vi "TetroInfoModulation.vi"(9 "TetroInfo Input":T1, 10 "GameCommand enum":T2, 11 "Playfield Input":bool[][](array[boolean])) -> (1 "TetroInfo Output":T1)   [LabVIEW 2026]
doc: "This VI i responsible for modifying an existing tetro info according to the users game commands"
uses:
  01_Typen/GameCommandTypeDef.ctl
  02_StateMachine/GameTetrominoInformationTypeDef.ctl
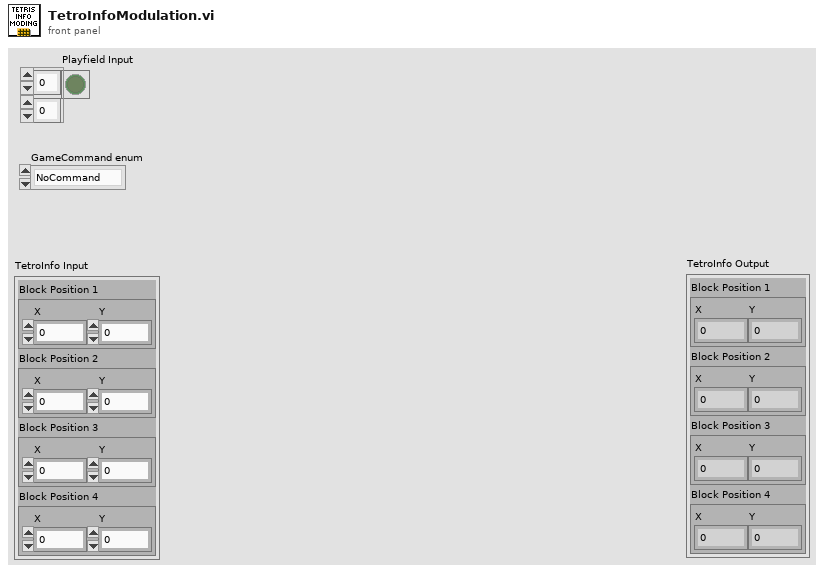
[diagram p1: front panel]
types:
  T1 = typedef "GameTetrominoInformationTypeDef.ctl" = cluster{"Block Position 1":cluster{"X":i32, "Y":i32}, "Block Position 2":cluster{"X":i32, "Y":i32}, "Block Position 3":cluster{"X":i32, "Y":i32}, "Block Position 4":cluster{"X":i32, "Y":i32}}
  T2 = typedef "GameCommandTypeDef.ctl" = enum16{"NoCommand", "Rotate", "MoveLeft", "MoveRight"}
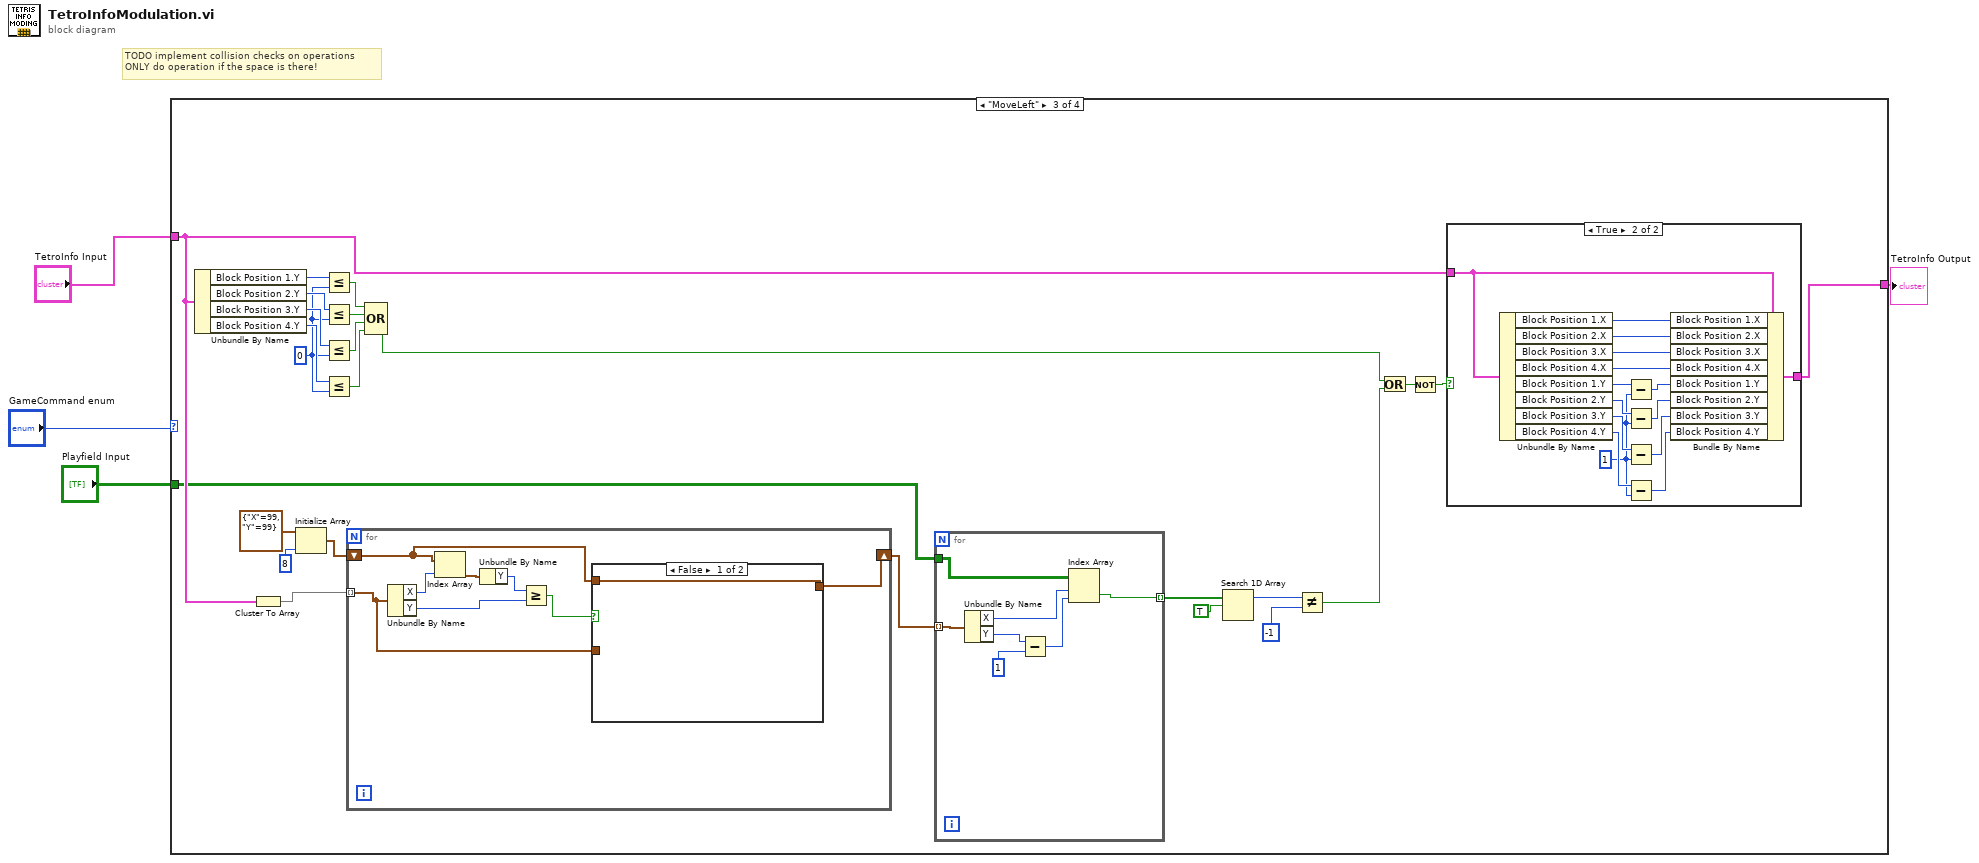
[diagram p0: block diagram]
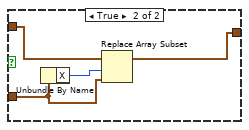
[diagram p4: hidden frame]
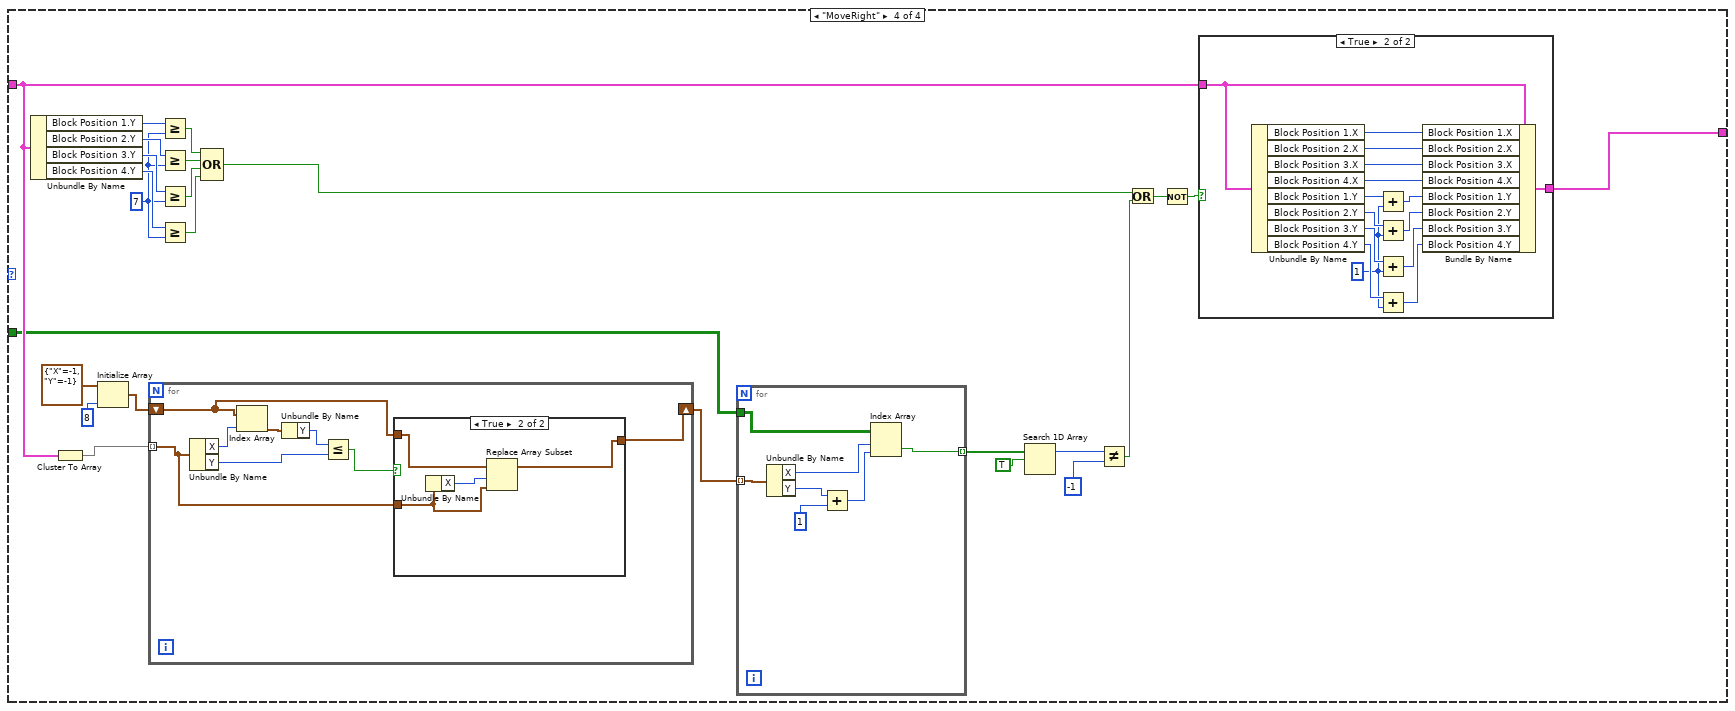
[diagram p6: hidden frame]
diagram:
  # "TODO implement collision checks on operations\nONLY do operation if the space is there!"
  n1 = case shown="\"MoveLeft\"" "GameCommand enum" {
    tunnel: "TetroInfo Input" -> [w5 w6 w9 w79]
    tunnel: [w5 w6 w19 w92] -> w2
    tunnel: "Playfield Input" -> [_ _ w8 w68]
    frame "NoCommand", Default {
    }
    frame "Rotate" {
      # "TODO implement rotate"
    }
    frame "MoveLeft" {
      w25 = 0 ("y")
      n2 = Unbundle By Name(w9) -> ("Block Position 1.Y"=w29:i32, "Block Position 2.Y"=w28:i32, "Block Position 3.Y"=w27:i32, "Block Position 4.Y"=w26:i32)
      n3 = Cluster To Array(cluster=w9) -> (array=w16:cluster{"X":i32, "Y":i32}[])
      n4 = Initialize Array(cluster{"X":i32, "Y":i32} {"X"=99, "Y"=99}, 8 ("dimension size")) -> (w15:cluster{"X":i32, "Y":i32}[])
      n5 = Less Or Equal?(x=w29, y=w25) -> (x <= y?=w23:bool)
      n6 = Less Or Equal?(x=w28, y=w25) -> (x <= y?=w22:bool)
      n7 = Less Or Equal?(x=w27, y=w25) -> (x <= y?=w21:bool)
      n8 = Less Or Equal?(x=w26, y=w25) -> (x <= y?=w20:bool)
      n9 = for {
        tunnel: w16 -> [w43] mode=indexing
        shift-right: [w41] -> w10
        shift-left: w15 -> [w42]
        n10 = Unbundle By Name(w43) -> ("X"=w46:i32, "Y"=w45:i32)
        n11 = Index Array(array=w42, index=w46) -> (element=w40:cluster{"X":i32, "Y":i32})
        n12 = Unbundle By Name(w40) -> ("Y"=w39:i32)
        n13 = Greater Or Equal?(x=w39, y=w45) -> (x >= y?=w44:bool)
        n14 = case shown="False" w44 {
          tunnel: w43 -> [_ w48]
          tunnel: w42 -> [w47 w51]
          tunnel: [w47 w50] -> w41
          frame False {
          }
          frame True {
            n15 = Unbundle By Name(w48) -> ("X"=w49:i32)
            n16 = Replace Array Subset(array=w51, new element=w48, index=w49) -> (w50:cluster{"X":i32, "Y":i32}[])
          }
        }
      }
      n17 = Compound Arithmetic op=OR(w23, w22, w21, w20) -> (w24:bool)
      n18 = for {
        tunnel: w10 -> [w38] mode=indexing
        tunnel: w8 -> [w37]
        tunnel: [w36] -> w11 mode=indexing
        n19 = Unbundle By Name(w38) -> ("X"=w35:i32, "Y"=w33:i32)
        n20 = Subtract(x=w33, y=1) -> (x-y=w34:i32)
        n21 = Index Array(array=w37, index (row)=w35, index (col)=w34) -> (element=w36:bool)
      }
      n22 = Search 1D Array(1D array=w11, element=TRUE) -> (index of element=w13:i32)  [unwired: 1 in]
      n23 = Not Equal?(x=w13, y=-1) -> (x != y?=w7:bool)
      n24 = Or(x=w24, y=w7) -> (x .or. y?=w30:bool)
      n25 = Not(x=w30) -> (.not. x?=w31:bool)
      n26 = case shown="True" w31 {
        tunnel: w9 -> [w52 w67]
        tunnel: [w52 w66] -> w19
        frame False {
        }
        frame True {
          w60 = 1 ("y")
          n27 = Unbundle By Name(w67) -> ("Block Position 1.X"=w56:i32, "Block Position 2.X"=w55:i32, "Block Position 3.X"=w54:i32, "Block Position 4.X"=w53:i32, "Block Position 1.Y"=w61:i32, "Block Position 2.Y"=w62:i32, "Block Position 3.Y"=w63:i32, "Block Position 4.Y"=w65:i32)
          n28 = Subtract(x=w61, y=w60) -> (x-y=w64:i32)
          n29 = Subtract(x=w62, y=w60) -> (x-y=w57:i32)
          n30 = Subtract(x=w63, y=w60) -> (x-y=w58:i32)
          n31 = Subtract(x=w65, y=w60) -> (x-y=w59:i32)
          n32 = Bundle By Name(cluster=w67, "Block Position 1.X"=w56, "Block Position 2.X"=w55, "Block Position 3.X"=w54, "Block Position 4.X"=w53, "Block Position 1.Y"=w64, "Block Position 2.Y"=w57, "Block Position 3.Y"=w58, "Block Position 4.Y"=w59) -> (w66:T1)
        }
      }
    }
    frame "MoveRight" {
      w85 = 7 ("y")
      n33 = Unbundle By Name(w79) -> ("Block Position 1.Y"=w89:i32, "Block Position 2.Y"=w88:i32, "Block Position 3.Y"=w87:i32, "Block Position 4.Y"=w86:i32)
      n34 = Cluster To Array(cluster=w79) -> (array=w76:cluster{"X":i32, "Y":i32}[])
      n35 = Initialize Array(cluster{"X":i32, "Y":i32} {"X"=-1, "Y"=-1}, 8 ("dimension size")) -> (w75:cluster{"X":i32, "Y":i32}[])
      n36 = for {
        tunnel: w76 -> [w104] mode=indexing
        shift-right: [w102] -> w69
        shift-left: w75 -> [w103]
        n37 = Unbundle By Name(w104) -> ("X"=w107:i32, "Y"=w106:i32)
        n38 = Index Array(array=w103, index=w107) -> (element=w101:cluster{"X":i32, "Y":i32})
        n39 = Unbundle By Name(w101) -> ("Y"=w100:i32)
        n40 = Less Or Equal?(x=w100, y=w106) -> (x <= y?=w105:bool)
        n41 = case shown="True" w105 {
          tunnel: w104 -> [_ w109]
          tunnel: w103 -> [w108 w112]
          tunnel: [w108 w111] -> w102
          frame False {
          }
          frame True {
            n42 = Unbundle By Name(w109) -> ("X"=w110:i32)
            n43 = Replace Array Subset(array=w112, new element=w109, index=w110) -> (w111:cluster{"X":i32, "Y":i32}[])
          }
        }
      }
      n44 = Greater Or Equal?(x=w89, y=w85) -> (x >= y?=w83:bool)
      n45 = Greater Or Equal?(x=w88, y=w85) -> (x >= y?=w82:bool)
      n46 = Greater Or Equal?(x=w87, y=w85) -> (x >= y?=w81:bool)
      n47 = Greater Or Equal?(x=w86, y=w85) -> (x >= y?=w80:bool)
      n48 = Compound Arithmetic op=OR(w83, w82, w81, w80) -> (w84:bool)
      n49 = for {
        tunnel: w69 -> [w99] mode=indexing
        tunnel: w68 -> [w98]
        tunnel: [w97] -> w71 mode=indexing
        n50 = Unbundle By Name(w99) -> ("X"=w96:i32, "Y"=w94:i32)
        n51 = Add(x=w94, y=1) -> (x+y=w95:i32)
        n52 = Index Array(array=w98, index (row)=w96, index (col)=w95) -> (element=w97:bool)
      }
      n53 = Search 1D Array(1D array=w71, element=TRUE) -> (index of element=w73:i32)  [unwired: 1 in]
      n54 = Not Equal?(x=w73, y=-1) -> (x != y?=w70:bool)
      n55 = Or(x=w84, y=w70) -> (x .or. y?=w90:bool)
      n56 = Not(x=w90) -> (.not. x?=w91:bool)
      n57 = case shown="True" w91 {
        tunnel: w79 -> [w113 w128]
        tunnel: [w113 w127] -> w92
        frame False {
        }
        frame True {
          w121 = 1 ("y")
          n58 = Unbundle By Name(w128) -> ("Block Position 1.X"=w117:i32, "Block Position 2.X"=w116:i32, "Block Position 3.X"=w115:i32, "Block Position 4.X"=w114:i32, "Block Position 1.Y"=w122:i32, "Block Position 2.Y"=w123:i32, "Block Position 3.Y"=w124:i32, "Block Position 4.Y"=w126:i32)
          n59 = Add(x=w122, y=w121) -> (x+y=w125:i32)
          n60 = Add(x=w123, y=w121) -> (x+y=w118:i32)
          n61 = Add(x=w124, y=w121) -> (x+y=w119:i32)
          n62 = Add(x=w126, y=w121) -> (x+y=w120:i32)
          n63 = Bundle By Name(cluster=w128, "Block Position 1.X"=w117, "Block Position 2.X"=w116, "Block Position 3.X"=w115, "Block Position 4.X"=w114, "Block Position 1.Y"=w125, "Block Position 2.Y"=w118, "Block Position 3.Y"=w119, "Block Position 4.Y"=w120) -> (w127:T1)
        }
      }
    }
  }
  "TetroInfo Output" <- w2
